vi "TipWarning.vi"() -> ()   [LabVIEW 2017]
panel:
  in  "Tip Warning":bool
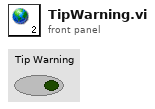
[diagram p1: front panel]
diagram:
